vi "readValueCommand.vi"(8 "error in (no error)":errorcluster, 11 "Tovey9150 in":refnum<class "Tovey9150.lvclass">) -> (0 "error out":errorcluster, 3 "Tovey9150 out":refnum<class "Tovey9150.lvclass">)   [LabVIEW 2015, in "Tovey9150.lvclass"]
uses:
  Tovey9150.lvclass
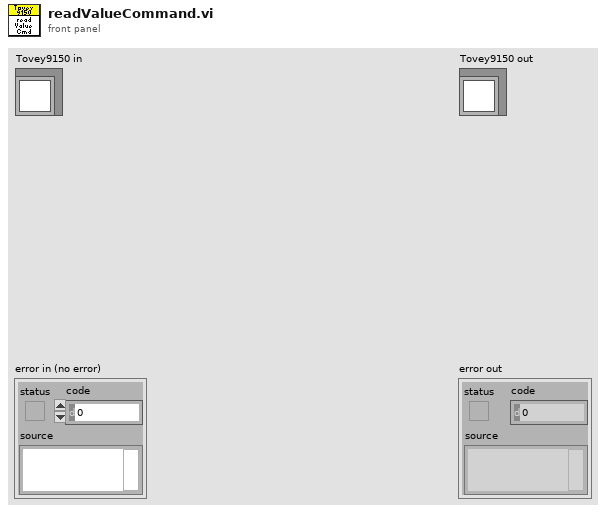
[diagram p1: front panel]
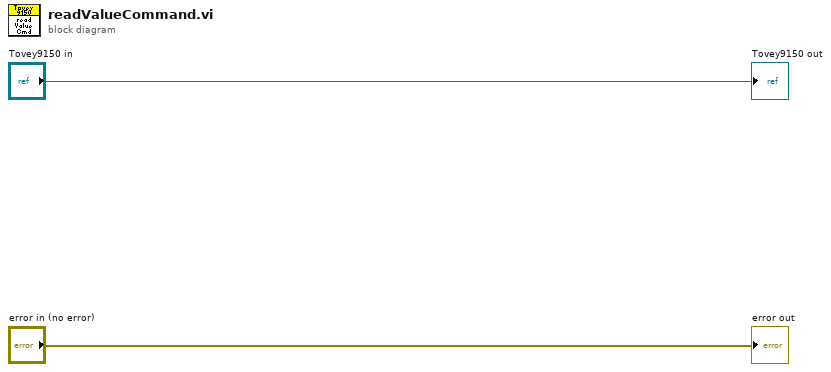
[diagram p0: block diagram]
diagram:
  "error out" <- "error in (no error)"
  "Tovey9150 out" <- "Tovey9150 in"
